vi "Command & Ack - Receive Ack.vi"(7 "Timeout (-1)":i32=-1, 8 "error in (no error)":errorcluster, 11 "SV B-M (Host) in":refnum<class "SV B-M (Host).lvclass">) -> (0 "error out":errorcluster, 1 "Message Data":variant, 2 "Message":string, 3 "SV B-M (Host) out":refnum<class "SV B-M (Host).lvclass">, 4 "Timeout?":bool)   [LabVIEW 2015, in "SV B-M (Host).lvclass"]
doc: "Wait on an acknowledgement from the target."
uses:
  SV B-M (Host).lvclass
  SV B-M (Host).lvclass/SV B-M (Host).ctl
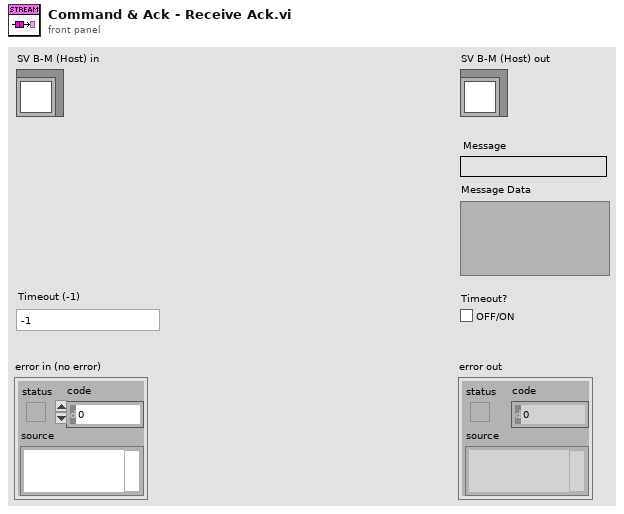
[diagram p1: front panel]
types:
  T1 = typedef "Message Cluster.ctl" = cluster{"Message":string, "Message Data":variant}
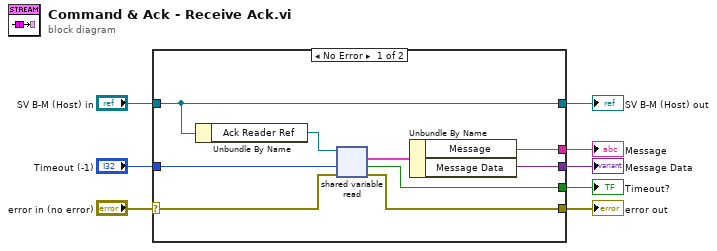
[diagram p0: block diagram]
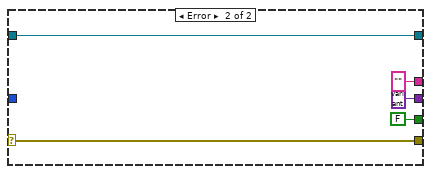
[diagram p2: hidden frame]
diagram:
  n1 = case shown="No Error" "error in (no error)" {
    selector: "error in (no error)" -> [w17 w22]
    tunnel: [w13 w22] -> w7
    tunnel: [w15 w21] -> w5
    tunnel: "SV B-M (Host) in" -> [w15 w21]
    tunnel: "Timeout (-1)" -> [w16 _]
    tunnel: [w11 "" ("Message")] -> w3
    tunnel: [w10 variant ("Message Data")] -> w2
    tunnel: [w9 FALSE] -> w1
    frame No Error {
      n2 = Unbundle By Name(w15) -> ("Ack Reader Ref"=w14:refnum<k21>)
      n3 = shared-variable-read(w14, w17, w16) -> (w13:errorcluster, w9:bool, w12:T1)  [unwired: 1 out]
      n4 = Unbundle By Name(w12) -> ("Message"=w11:string, "Message Data"=w10:variant)
    }
    frame Error {
    }
  }
  "error out" <- w7
  "SV B-M (Host) out" <- w5
  "Message" <- w3
  "Message Data" <- w2
  "Timeout?" <- w1
